vi "from string.vi"(8 "error in":errorcluster, 9 "data":string, 10 "version":string, 11 "configuration in":refnum<class "Bus Configuration.lvclass">) -> (0 "error out":errorcluster, 3 "configuration out":refnum<class "Bus Configuration.lvclass">)   [LabVIEW 2014, in "Bus Configuration.lvclass"]
doc: "Provides an interface for loading a module configuration from a file or other serialized data source. It is recommended that all children of this class store data in two sets--data required for its own initialization, and any data required for parent initialization--and that each implementation uses the <b>Call Parent Method</b> primitive to de-serialize parent information."
uses:
  Bus Configuration.lvclass
  SPI Configuration.ctl
  Bus Configuration.lvclass/Bus Configuration.ctl
  <vilib>/NI/Configuration Framework/serializable configuration/NISE_CEF_serializable configuration.lvclass
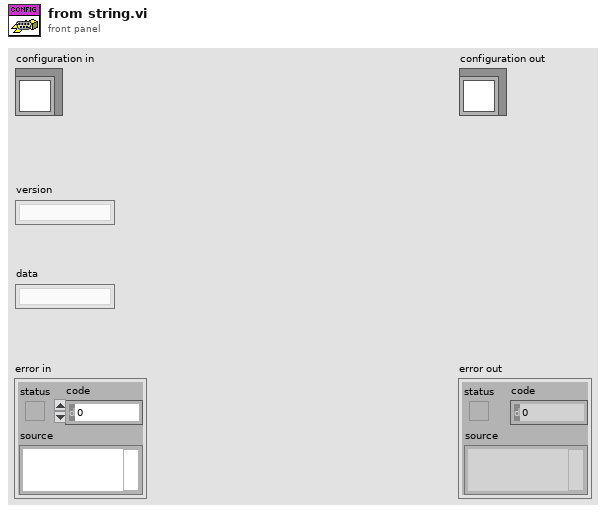
[diagram p1: front panel]
types:
  T1 = typedef "Bus Configuration.lvclass/SPI Configuration.ctl" = cluster{"SCLK":string, "MOSI":string, "MISO":string}
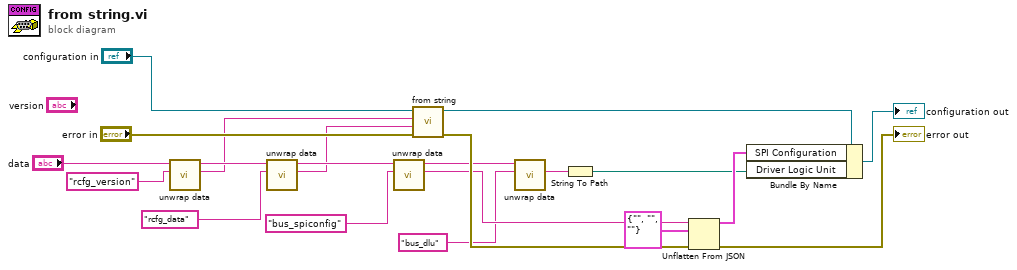
[diagram p0: block diagram]
diagram:
  n1 = call <vilib>:"unwrap data.vi"("identifier"="rcfg_version" ("additional identifier"), "data to unwrap"="data") -> ("unwrapped data"=w12:string, "remaining string"=w18:string)  [unwired: 8 in]
  n2 = call <vilib>:"unwrap data.vi"("identifier"="rcfg_data" ("additional identifier"), "data to unwrap"=w18) -> ("unwrapped data"=w11:string, "remaining string"=w16:string)  [unwired: 8 in]
  n3 = call <vilib>:"unwrap data.vi"("identifier"="bus_spiconfig" ("additional identifier"), "data to unwrap"=w16) -> ("unwrapped data"=w5:string, "remaining string"=w4:string)  [unwired: 8 in]
  n4 = call-parent "from string.vi"("error in"="error in", "data"=w11, "version"=w12, "configuration in"="configuration in") -> ("error out"=w8:errorcluster, "configuration out"=w10:refnum<class "Bus Configuration.lvclass">)  [unwired: 6 in]
  n5 = call <vilib>:"unwrap data.vi"("identifier"="bus_dlu", "data to unwrap"=w4) -> ("unwrapped data"=w3:string)  [unwired: 8 in, 1 out]
  n6 = String To Path(string=w3) -> (path=w2:path)
  n7 = Unflatten From JSON(JSON string=w5, type and defaults=T1 {"SCLK"="", "MOSI"="", "MISO"=""} ("SPI Configuration"), error in (no error)=w8) -> (value=w9:T1, error out=→"error out":errorcluster)  [unwired: 4 in]
  n8 = Bundle By Name(cluster=w10, "SPI Configuration"=w9, "Driver Logic Unit"=w2) -> (→"configuration out":refnum<class "Bus Configuration.lvclass">)
